vi "GetMaxRecordLength.vi"(8 "error in (no error)":errorcluster) -> (0 "error out":errorcluster, 3 "function return":i32)   [LabVIEW 2013, in "HS3OverallRoutines.lvlib"]
doc: "The different instruments have different record lengths. This\nroutine queries the maximum available record length per channel, in samples.\n\nInput: -\nOutput: Return value The maximum record length the instrument supports, in number of samples\n\nint GetMaxRecordLength ( void );"
uses:
  HS3OverallRoutines.lvlib
  hs3.dll
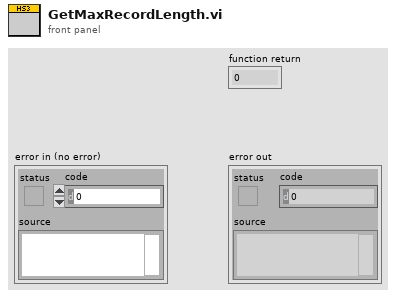
[diagram p1: front panel]
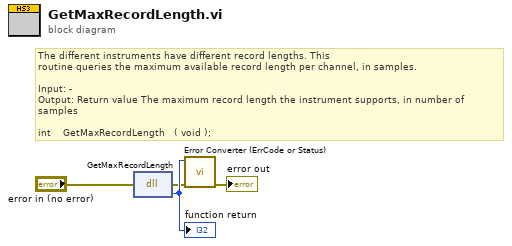
[diagram p0: block diagram]
diagram:
  # "The different instruments have different record lengths. This\nroutine queries the maximum available record length per channel, in samples.\n\nInput: -\nOutput: Return value The maximum record length the instrument supports, in number of samples\n\nint \t\t\tGetMaxRecordLength\t\t\t( void );"
  n1 = dll-call lib="C:/Documents and Settings/admin/Pulpit/HS3 LabViewLib/HS3_WRAPPER/OverallRoutines/hs3.*" fn="GetMaxRecordLength"(error in="error in (no error)") -> (error out=w2:errorcluster, w4:i32)  [unwired: 2 in, 1 out]
  "function return" <- w4
  n2 = call "Error Converter (ErrCode or Status).vi"("error in (no error)"=w2, "error code"=w4) -> ("error out"=→"error out":errorcluster)  [unwired: 9 in]
